vi "Polynomial GCD Pair (DBL).vi"(9 "tolerance":dbl=1e-08, 10 "Q(x)":dbl[](array[numeric]), 11 "P(x)":dbl[](array[numeric])) -> (0 "error":i32, 1 "Co-factor of Q(x)":dbl[](array[numeric]), 2 "Co-factor of P(x)":dbl[](array[numeric]), 3 "Greatest Common Divisor":dbl[](array[numeric]))   [LabVIEW 2020, in "NI_AALPro.lvlib"]
uses:
  <vilib>/Analysis/NI_AALPro.lvlib
  <resource>/lvanlys.dll
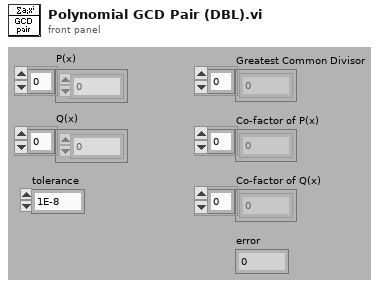
[diagram p1: front panel]
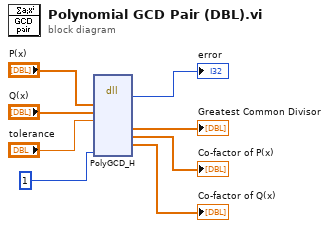
[diagram p0: block diagram]
diagram:
  n1 = dll-call lib="e:/builds/penguin/labview/branches/2020/dev/dist/resource/lvanlys.*" fn="PolyGCD_H"("P"="P(x)", "Q"="Q(x)", "tol"="tolerance", "isLCM"=1) -> (→"error":i32, "U"=→"Greatest Common Divisor":dbl[], "V"=→"Co-factor of P(x)":dbl[], "W"=→"Co-factor of Q(x)":dbl[])  [unwired: 10 in, 2 out]
